vi "TcA01-004_ObjectCreationAndDestructionWithDefaultConstructor.vi"(1 "Input buffer":T3="1", 3 "Invocation info":T2, 5 "error in (no error)":errorcluster, 6 "Add log to result?":bool) -> (16 "Test Data":T1 {"Numeric Measurement" format="%.2f"}, 19 "error out":errorcluster)   [LabVIEW 2020]
doc: "Test case template."
uses:
  Shared/Support_InputBuffer.ctl
  Shared/Support_InvocationInfo.ctl
  Shared/Support_TestData.ctl
  TestClasses/G#SubSubClass1_class/G#SubSubClass1.lvclass
  C:/Program Files (x86)/National Instruments/LabVIEW 2020/vi.lib/addons/_AddQ/G#Object/G#Object.lvclass
  TestClasses/G#SubClass1_class/G#SubClass1.lvclass
  TestClasses/G#BaseClass1_class/G#BaseClass1.lvclass
  TestClasses/G#BaseAggregator_class/G#BaseAggregator.lvclass
  <vilib>/addons/_AddQ/G#Object/G#Object.lvclass
panel:
  in  "Test name":string="TcA01-004 Object creation and destruction with default constructor"
  out "Test result":bool
  out "Result":string
  # "Verify that multiple objects of a base class can\nbe created and destructed multiple times."
  # "Sub test case"
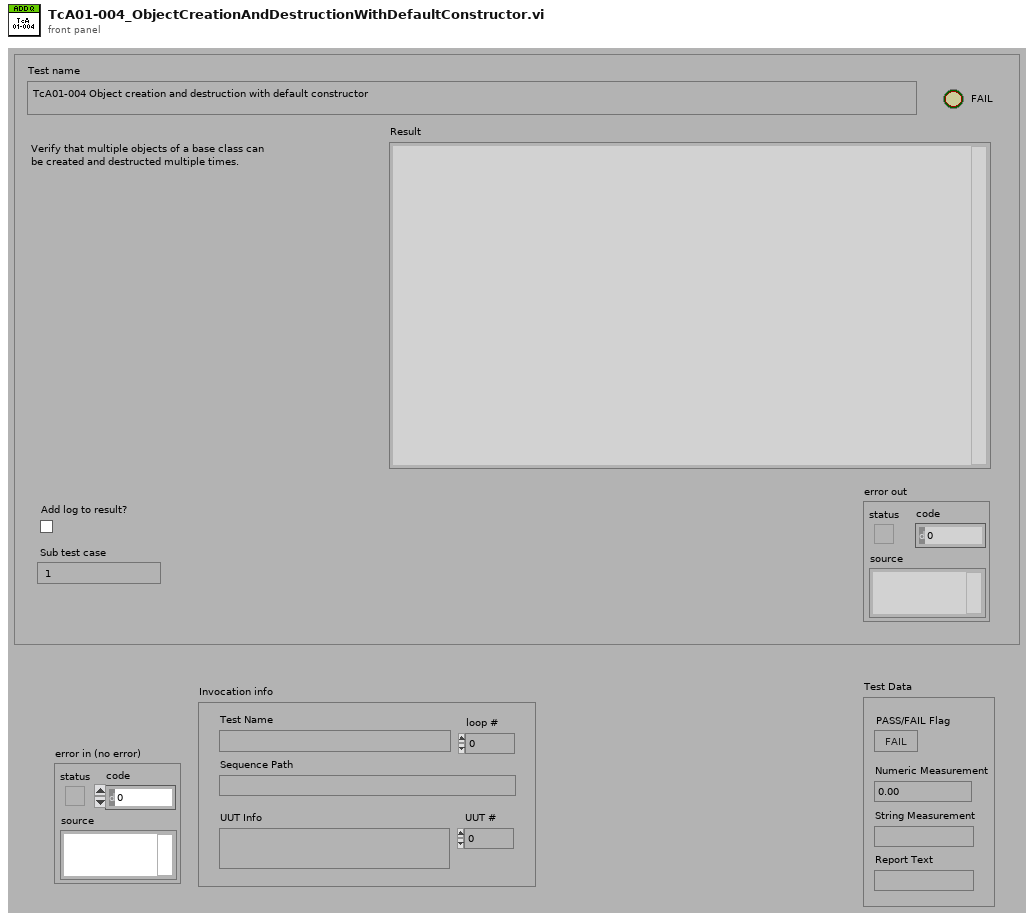
[diagram p1: front panel]
types:
  T1 = typedef "Support_TestData.ctl" = cluster{"PASS/FAIL Flag":bool, "Numeric Measurement":dbl, "String Measurement":string, "Report Text":string}
  T2 = typedef "Support_InvocationInfo.ctl" = cluster{"UUT #":i32, "loop #":i32, "UUT Info":string, "Test Name":string, "Sequence Path":path}
  T3 = typedef "Support_InputBuffer.ctl" = string
  T4 = typedef "Support_ResultType.ctl" = cluster{"Pass":bool, "Comment":string, "MeasurementValue":dbl}
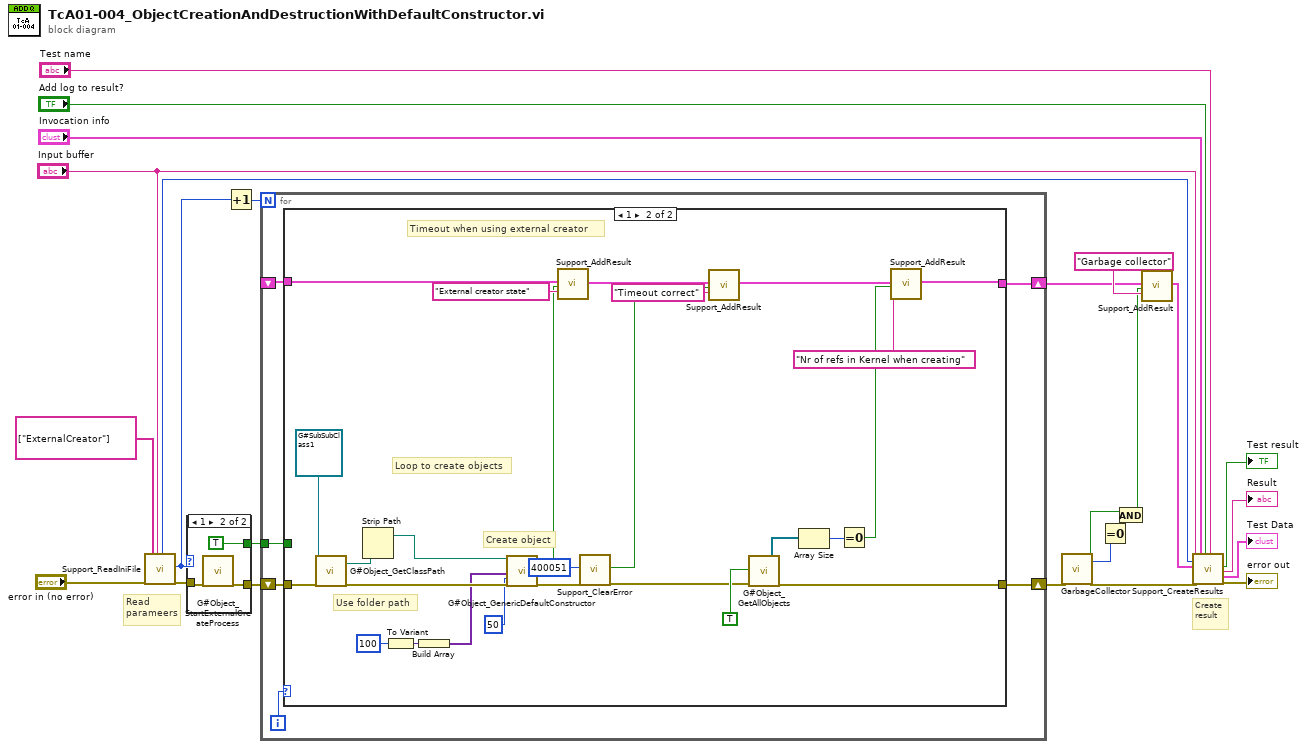
[diagram p0: block diagram]
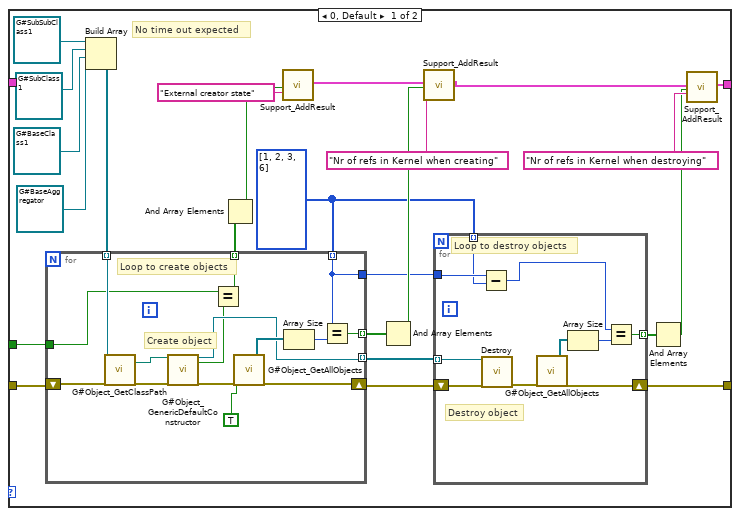
[diagram p2: hidden frame]
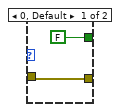
[diagram p3: hidden frame]
diagram:
  # "Read\nparameers"
  # "Create\nresult"
  n1 = call "Support_ReadIniFile.vi"("error in (no error)"="error in (no error)", "Parameter names"=string[] ["ExternalCreator"], "Sub test case"="Input buffer") -> ("Timer start"=w16:u32, "Parameter1 as I32"=w1:i32, "error out"=w7:errorcluster)  [unwired: 9 in, 5 out]
  n2 = case shown="1" w1 {
    tunnel: w7 -> [w27 w30]
    tunnel: [w27 w29] -> w6
    tunnel: [FALSE TRUE] -> w4
    frame 0, Default {
    }
    frame 1 {
      n3 = call <vilib>:"G#Object_StartExternalCreateProcess.vi"("error in (no error)"=w30) -> ("error out"=w29:errorcluster)  [unwired: 18 in]
    }
  }
  n4 = Increment(x=w1) -> (x+1=w2:i32)
  n5 = for {
    N: w2 -> [_]
    tunnel: w4 -> [w33]
    shift-right: [w36] -> w15
    shift-left: w6 -> [w35]
    shift-right: [w34] -> w5
    shift-left: _ -> [w31]
    i -> [w32]
    n6 = case shown="1" w32 {
      tunnel: [w52 w100] -> w36
      tunnel: w35 -> [w50 w110]
      tunnel: [w43 w99] -> w34
      tunnel: w33 -> [w40 _]
      tunnel: w31 -> [_ w86]
      frame 0, Default {
        w46 = i32[] [1, 2, 3, 6]
        # "No time out expected"
        n7 = Build Array(refnum<class "G#SubSubClass1.lvclass"> refnum ("G#SubSubClass1.lvclass"), refnum<class "G#SubClass1.lvclass"> refnum ("G#SubClass1.lvclass"), refnum<class "G#BaseClass1.lvclass"> refnum ("G#BaseClass1.lvclass"), refnum<class "G#BaseAggregator.lvclass"> refnum ("G#BaseAggregator.lvclass")) -> (w44:refnum<class "G#Object.lvclass">[])
        n8 = for {
          shift-right: [w80] -> w57
          shift-left: w50 -> [w78]
          tunnel: [w79] -> w51 mode=indexing
          tunnel: [w84] -> w60 mode=indexing
          tunnel: w44 -> [w76] mode=indexing
          tunnel: w46 -> [w74] mode=indexing
          tunnel: [w74] -> w45
          tunnel: w40 -> [w72]
          tunnel: [w71] -> w39 mode=indexing
          # "Create object"
          # "Loop to create objects"
          n9 = call-dynamic "G#Object_GetClassPath.vi"("reference in"=w76, "error in (no error)"=w78) -> ("class path"=w75:path, "error out"=w77:errorcluster)  [unwired: 15 in, 1 out]
          n10 = call <vilib>:"G#Object_GenericDefaultConstructor.vi"("class path"=w75, "error in (no error)"=w77) -> ("reference out"=w79:refnum<class "G#Object.lvclass">, "external creator running?"=w73:bool, "error out"=w83:errorcluster)  [unwired: 15 in]
          n11 = Equal?(x=w72, y=w73) -> (x = y?=w71:bool)
          n12 = call <vilib>:"G#Object_GetAllObjects.vi"("only refs (F)"=TRUE ("only refs"), "error in (no error)"=w83) -> ("all refs"=w82:refnum<class "G#Object.lvclass">[], "error out"=w80:errorcluster)  [unwired: 14 in, 2 out]
          n13 = Array Size(array=w82) -> (size(s)=w85:i32)
          n14 = Equal?(x=w74, y=w85) -> (x = y?=w84:bool)
        }
        n15 = And Array Elements(Boolean array=w39) -> (logical AND=w38:bool)
        n16 = call "Support_AddResult.vi"("Pass"=w38, "Comment"="External creator state") -> ("Results out"=w41:T4[])  [unwired: 17 in]
        n17 = And Array Elements(Boolean array=w60) -> (logical AND=w58:bool)
        n18 = call "Support_AddResult.vi"("Results in"=w41, "Pass"=w58, "Comment"="Nr of refs in Kernel when creating") -> ("Results out"=w53:T4[])  [unwired: 16 in]
        n19 = for {
          shift-right: [w61] -> w52
          shift-left: w57 -> [w69]
          tunnel: [w70] -> w56 mode=indexing
          tunnel: w51 -> [w66] mode=indexing
          tunnel: w45 -> [w68]
          tunnel: w46 -> [w62] mode=indexing
          # "Destroy object"
          # "Loop to destroy objects"
          n20 = Subtract(x=w68, y=w62) -> (x-y=w67:i32)
          n21 = call-dynamic "Destroy.vi"("reference in"=w66, "error in (no error)"=w69) -> ("error out"=w63:errorcluster)  [unwired: 16 in, 1 out]
          n22 = call <vilib>:"G#Object_GetAllObjects.vi"("error in (no error)"=w63) -> ("all refs"=w64:refnum<class "G#Object.lvclass">[], "error out"=w61:errorcluster)  [unwired: 15 in, 2 out]
          n23 = Array Size(array=w64) -> (size(s)=w65:i32)
          n24 = Equal?(x=w67, y=w65) -> (x = y?=w70:bool)
        }
        n25 = And Array Elements(Boolean array=w56) -> (logical AND=w54:bool)
        n26 = call "Support_AddResult.vi"("Results in"=w53, "Pass"=w54, "Comment"="Nr of refs in Kernel when destroying") -> ("Results out"=w43:T4[])  [unwired: 16 in]
      }
      frame 1 {
        # "Use folder path"
        # "Create object"
        # "Loop to create objects"
        # "Timeout when using external creator"
        n27 = call-dynamic "G#Object_GetClassPath.vi"("reference in"=refnum<class "G#SubSubClass1.lvclass"> refnum ("G#SubSubClass1.lvclass"), "error in (no error)"=w110) -> ("class path"=w104:path, "error out"=w106:errorcluster)  [unwired: 15 in, 1 out]
        n28 = Strip Path(path=w104) -> (stripped path=w103:path)  [unwired: 1 out]
        n29 = To Variant(anything=100 ("timeout (ms)")) -> (Variant=w93:variant)
        n30 = Build Array(w93) -> (w92:variant[])
        n31 = call <vilib>:"G#Object_GenericDefaultConstructor.vi"("class path"=w103, "control values"=w92, "timeout in ms (-1)"=50 ("timeout (ms)"), "error in (no error)"=w106) -> ("external creator running?"=w98:bool, "error out"=w91:errorcluster)  [unwired: 13 in, 1 out]
        n32 = call "Support_AddResult.vi"("Results in"=w86, "Pass"=w98, "Comment"="External creator state") -> ("Results out"=w97:T4[])  [unwired: 16 in]
        n33 = call "Support_ClearError.vi"("code"=400051, "error in (no error)"=w91) -> ("Cleared?"=w88:bool, "error out"=w90:errorcluster)  [unwired: 16 in]
        n34 = call "Support_AddResult.vi"("Results in"=w97, "Pass"=w88, "Comment"="Timeout correct") -> ("Results out"=w96:T4[])  [unwired: 16 in]
        n35 = call <vilib>:"G#Object_GetAllObjects.vi"("only refs (F)"=TRUE ("only refs"), "error in (no error)"=w90) -> ("all refs"=w108:refnum<class "G#Object.lvclass">[], "error out"=w100:errorcluster)  [unwired: 14 in, 2 out]
        n36 = Array Size(array=w108) -> (size(s)=w102:i32)
        n37 = Equal To 0?(x=w102) -> (x = 0?=w101:bool)
        n38 = call "Support_AddResult.vi"("Results in"=w96, "Pass"=w101, "Comment"="Nr of refs in Kernel when creating") -> ("Results out"=w99:T4[])  [unwired: 16 in]
      }
    }
  }
  n39 = call <vilib>:"GarbageCollector.vi"("error in (no error)"=w15) -> ("OK"=w11:bool, "# of objects killed"=w9:i32, "error out"=w14:errorcluster)  [unwired: 16 in]
  n40 = Equal To 0?(x=w9) -> (x = 0?=w10:bool)
  n41 = And(x=w11, y=w10) -> (x .and. y?=w8:bool)
  n42 = call "Support_AddResult.vi"("Results in"=w5, "Pass"=w8, "Comment"="Garbage collector") -> ("Results out"=w13:T4[])  [unwired: 16 in]
  n43 = call "Support_CreateResults.vi"("Sub test case"="Input buffer", "Timer start"=w16, "Results"=w13, "error in (no error)"=w14, "Invocation info"="Invocation info", "Add log to result?"="Add log to result?", "Test name"="Test name") -> ("Pass/fail flag"=→"Test result":bool, "Result"=→"Result":string, "Test Data"=→"Test Data":T1, "error out"=→"error out":errorcluster)  [unwired: 9 in]
